vi "__MergeVAttributes.vi"(6 "If exist? Skip(T)/Overwrite(F)":bool, 8 "error in (no error)":errorcluster, 10 "VAttributes B":variant, 11 "VAttributes A":variant) -> (0 "error out":errorcluster, 3 "VAttributes A after B->A":variant)   [LabVIEW 2019, in "lv-apt-json-file.lvlib"]
uses:
  lv-apt-json-file.lvlib
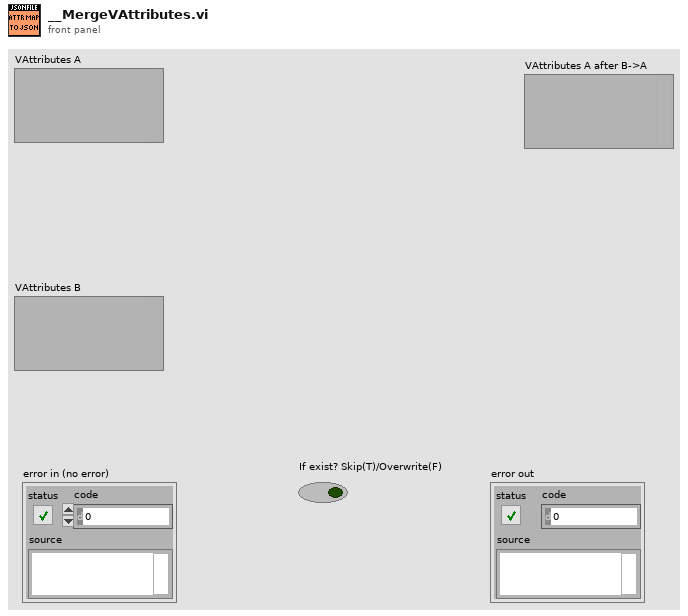
[diagram p1: front panel]
types:
  T1 = typedef "Type Descriptor Enumeration__ogtk.ctl" = enum8{"<Null>", "I8", "I16", "I32", "I64", "U8", "U16", "U32", "U64", "SGL", "DBL", "EXT", "CSG", "CDB", "CXT", "0x0F", "0x10", "0x11", "0x12", "0x13", "0x14", "Enum U8", "Enum U16", "Enum U32", "Enum U64", "SGL PQ", "DBL PQ", "EXT PQ", "CSG PQ", "CDB PQ", "CXT PQ", "0x1F", "0x20", "Boolean", "0x22", "0x23", "0x24", "0x25", "0x26", "0x27", "0x28", "0x29", "0x2A", "0x2B", "0x2C", "0x2D", "0x2E", "0x2F", "String", "0x31", "Path", "Pict", "0x34", "0x35", "0x36", "DAQ", "0x38", "0x39", "0x3A", "0x3B", "0x3C", "0x3D", "0x3E", "0x3F", "Array", "0x41", "0x42", "0x43", "0x44", "0x45", "0x46", "0x47", "0x48", "0x49", "0x4A", "0x4B", "0x4C", "0x4D", "0x4E", "0x4F", "Cluster", "0x51", "0x52", "Variant", "Waveform", "0x55", "0x56", "0x57", "0x58", "0x59", "0x5A", "0x5B", "0x5C", "0x5D", "0x5E", "0x5F", "0x60", "0x61", "0x62", "0x63", "0x64", "0x65", "0x66", "0x67", "0x68", "0x69", "0x6A", "0x6B", "0x6C", "0x6D", "0x6E", "0x6F", "Refnum"}
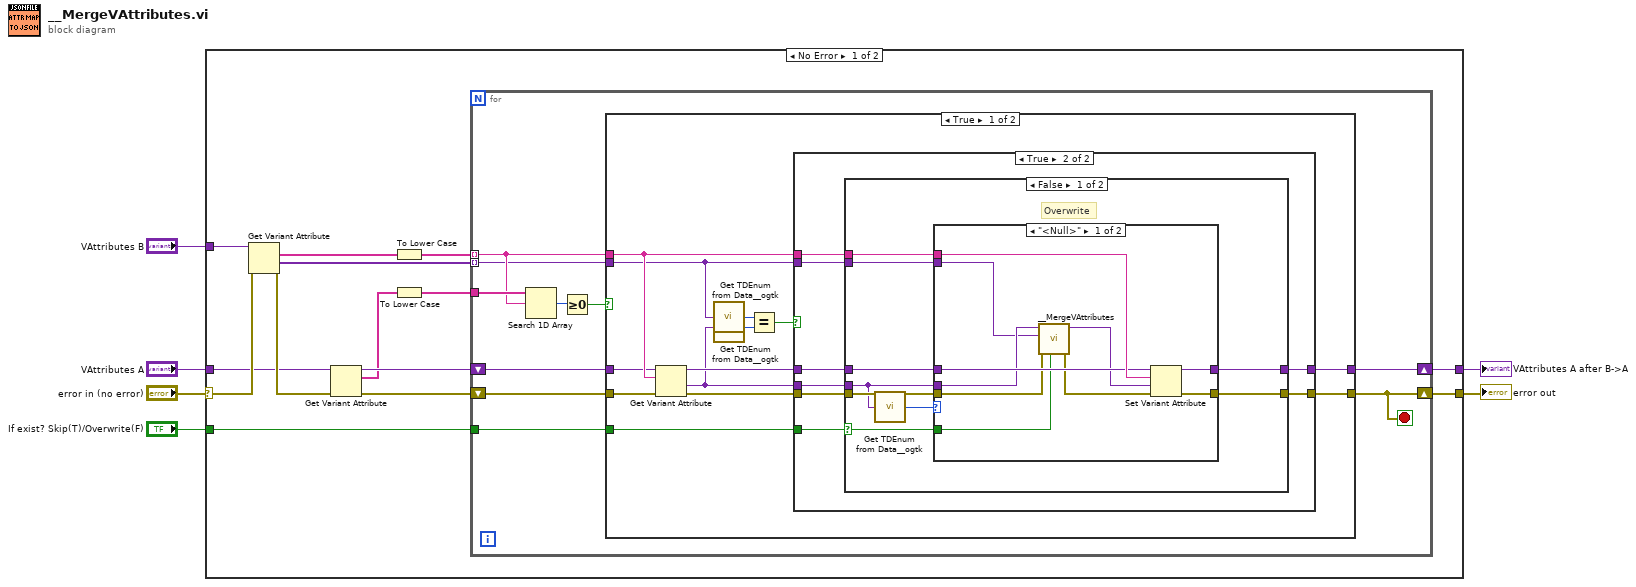
[diagram p0: block diagram]
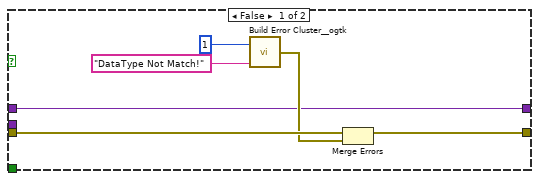
[diagram p2: hidden frame]
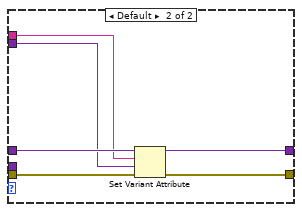
[diagram p3: hidden frame]
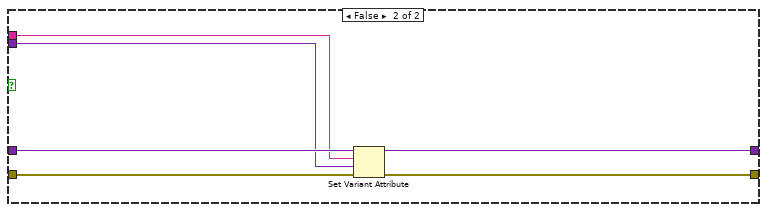
[diagram p5: hidden frame]
diagram:
  n1 = case shown="No Error" "error in (no error)" {
    selector: "error in (no error)" -> [w17 w92]
    tunnel: "VAttributes A" -> [w11 w91]
    tunnel: "VAttributes B" -> [w12 _]
    tunnel: "If exist? Skip(T)/Overwrite(F)" -> [w7 _]
    tunnel: [w9 w92] -> w2
    tunnel: [w10 w91] -> w1
    frame No Error {
      n2 = Get Variant Attribute(Variant=w12, error in=w17) -> (names=w14:string[], values=w15:variant[], error out=w16:errorcluster)  [unwired: 2 in, 1 out]
      n3 = Get Variant Attribute(Variant=w11, error in=w16) -> (duplicate Variant=w20:variant, names=w19:string[], error out=w8:errorcluster)  [unwired: 2 in, 1 out]
      n4 = To Lower Case(string=w14) -> (all lower case string=w13:string[])
      n5 = To Lower Case(string=w19) -> (all lower case string=w18:string[])
      n6 = for {
        shift-right: [w29] -> w10
        shift-left: w20 -> [w30]
        shift-right: [w21] -> w9
        shift-left: w8 -> [w28]
        tunnel: w18 -> [w27]
        tunnel: w15 -> [w23] mode=indexing
        tunnel: w13 -> [w24] mode=indexing
        tunnel: w7 -> [w22]
        stop <- w21 stop-if-true
        n7 = Search 1D Array(1D array=w27, element=w24) -> (index of element=w26:i32)  [unwired: 1 in]
        n8 = Greater Or Equal To 0?(x=w26) -> (x >= 0?=w25:bool)
        n9 = case shown="True" w25 {
          tunnel: w30 -> [w38 w90]
          tunnel: [w43 w89] -> w29
          tunnel: w28 -> [w42 w88]
          tunnel: [w41 w87] -> w21
          tunnel: w24 -> [w40 w86]
          tunnel: w23 -> [w35 w85]
          tunnel: w22 -> [w37 _]
          frame True {
            n10 = Get Variant Attribute(Variant=w38, name=w40, error in=w42) -> (duplicate Variant=w39:variant, value=w34:variant, error out=w36:errorcluster)  [unwired: 1 in, 1 out]
            n11 = call <userlib>:"Get TDEnum from Data__ogtk.vi"("Data"=w35) -> ("Type Descriptor Enumeration"=w32:T1)  [unwired: 4 in]
            n12 = call <userlib>:"Get TDEnum from Data__ogtk.vi"("Data"=w34) -> ("Type Descriptor Enumeration"=w33:T1)  [unwired: 4 in]
            n13 = Equal?(x=w32, y=w33) -> (x = y?=w31:bool)
            n14 = case shown="True" w31 {
              tunnel: [w44 w57] -> w43
              tunnel: [w49 w56] -> w41
              tunnel: w40 -> [_ w55]
              tunnel: w39 -> [w44 w54]
              tunnel: w37 -> [_ w53]
              tunnel: w36 -> [w48 w52]
              tunnel: w35 -> [_ w51]
              tunnel: w34 -> [_ w50]
              frame False {
                n15 = call <userlib>:"Build Error Cluster__ogtk.vi"("String to Prepend to source (\"\")"="DataType Not Match!" ("String to Prepend to source (\"\")"), "code"=1) -> ("error out"=w47:errorcluster)
                n16 = Merge Errors(w48, w47) -> (w49:errorcluster)
              }
              frame True {
                n17 = case shown="False" w53 {
                  selector: w53 -> [w58 _]
                  tunnel: [w66 w84] -> w57
                  tunnel: [w65 w83] -> w56
                  tunnel: w55 -> [w64 _]
                  tunnel: w54 -> [w63 w84]
                  tunnel: w52 -> [w62 w83]
                  tunnel: w51 -> [w61 _]
                  tunnel: w50 -> [w60 _]
                  frame False {
                    # "Overwrite"
                    n18 = call <userlib>:"Get TDEnum from Data__ogtk.vi"("Data"=w60) -> ("Type Descriptor Enumeration"=w59:T1)  [unwired: 4 in]
                    n19 = case shown="\"<Null>\"" w59 {
                      tunnel: [w76 w81] -> w66
                      tunnel: [w75 w77] -> w65
                      tunnel: w64 -> [w74 w79]
                      tunnel: w63 -> [w73 w82]
                      tunnel: w61 -> [w71 w78]
                      tunnel: w60 -> [w72 _]
                      tunnel: w62 -> [w70 w80]
                      tunnel: w58 -> [w67 _]
                      frame "<Null>" {
                        n20 = call "__MergeVAttributes.vi"("If exist? Skip(T)/Overwrite(F)"=w67, "error in (no error)"=w70, "VAttributes B"=w71, "VAttributes A"=w72) -> ("error out"=w69:errorcluster, "VAttributes A after B->A"=w68:variant)  [unwired: 6 in]
                        n21 = Set Variant Attribute(Variant=w73, name=w74, value=w68, error in=w69) -> (Variant out=w76:variant, error out=w75:errorcluster)  [unwired: 1 out]
                      }
                      frame Default {
                        n22 = Set Variant Attribute(Variant=w82, name=w79, value=w78, error in=w80) -> (Variant out=w81:variant, error out=w77:errorcluster)  [unwired: 1 out]
                      }
                    }
                  }
                  frame True {
                    # "Skip"
                  }
                }
              }
            }
          }
          frame False {
            n23 = Set Variant Attribute(Variant=w90, name=w86, value=w85, error in=w88) -> (Variant out=w89:variant, error out=w87:errorcluster)  [unwired: 1 out]
          }
        }
      }
    }
    frame Error {
    }
  }
  "error out" <- w2
  "VAttributes A after B->A" <- w1
